vi "AG33XXX.set DC offset.vi"(0 "i ref in":refnum<vi>, 2 "DCOffset [V]":dbl, 3 "ms timeout (10000)":i32=10000, 5 "error in (no error)":errorcluster) -> (14 "i ref out":refnum<vi>, 17 "timed out":bool, 19 "error out":errorcluster)   [LabVIEW 2014, in "AG33XXX.lvlib"]
doc: "Sets the DC offset at my device."
uses:
  AG33XXX.lvlib
  CSCore/CSApplicationBaseClasses/AFGBase/AFGBase.serviceType.ctl
  CSCore/CSApplicationBaseClasses/AFGBase/AFGBase.directionType.ctl
  CSlibraries/UtilityLib/UtilityLib.valueStatus.ctl
  CSCore/CSApplicationBaseClasses/DeviceBase/DeviceBase.lvlib
  CSCore/CSApplicationBaseClasses/AFGBase/AFGBase.lvlib
  CSlibraries/UtilityLib/UtilityLib.lvlib
  CSinstr.lib/Agilent 33xxx Series/Agilent 33XXX Series.lvlib
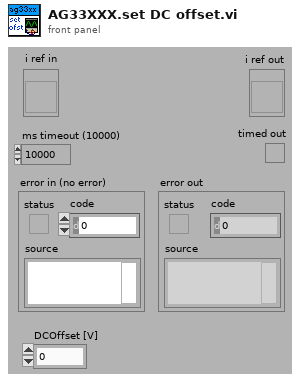
[diagram p1: front panel]
types:
  T1 = typedef "UtilityLib.lvlib/UtilityLib.valueStatus.ctl" = enum16{"no info available", "stand by/off", "on", "warning", "alarm/malfunction", "not implemented", "user action required", "important information", "system default", "control default", "indicator default", "button default"}
  T2 = typedef "AFGBase.lvlib/AFGBase.directionType.ctl" = enum16{"unknown", "update actual value", "update nominal value", "update both"}
  T3 = typedef "AFGBase.lvlib/AFGBase.serviceType.ctl" = enum16{"frequency", "amplitude", "phase", "DCOffset", "enableOutput", "trigger", "waveformType"}
  T4 = typedef "AFGBase.lvlib/AFGBase.i attribute.ctl" = cluster{"actValues":T5, "nomValues":T5}
  T5 = typedef "AFGBase.lvlib/AFGBase.parameters.ctl" = cluster{"frequency":dbl, "amplitude":dbl, "phase":dbl, "DCOffset":dbl, "waveformType":T6, "enableOutput":bool, "trigger":i16[], "serviceIDs":cluster{"frequencyID":i32, "amplitudeID":i32, "phaseID":i32, "DCOffsetID":i32, "waveformTypeID":i32, "enableOutputID":i32, "triggerID":i32}, "waveform":cluster{"data":waveform(dbl), "gain":dbl, "offset":dbl, "repetitionRate":dbl, "sampleRate":dbl}}
  T6 = typedef "AFGBase.lvlib/AFGBase.waveformType.ctl" = enum16{"sine", "square", "ramp", "pulse", "noise", "DC", "arbitrary", "triangle", "ramp_up", "ramp_down", "amplitude modulation"}
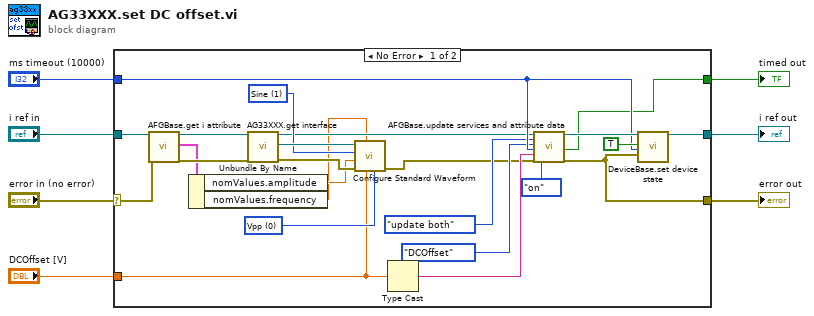
[diagram p0: block diagram]
diagram:
  n1 = case shown="No Error" "error in (no error)" {
    selector: "error in (no error)" -> [w20 w32]
    tunnel: [w31 w33] -> w7
    tunnel: "ms timeout (10000)" -> [w27 _]
    tunnel: "i ref in" -> [w21 w33]
    tunnel: [w28 w32] -> w3
    tunnel: "DCOffset [V]" -> [w10 _]
    tunnel: [w8 _] -> w1
    frame No Error {
      w13 = u16 0 items=["Vpp", "Vrms", "dB"] ("Unit (0: Vpp)")
      w15 = u16 1 items=["DC", "Sine", "Square", "Triangle", "Ramp", "Pulse", "Noise", "Sinc", "Negative Ramp", "Exponential Rise", "Exponential Fall", "Cardiac"] ("Waveform Function (1: Sine)")
      n2 = call "AFGBase.get i attribute.vi"("i ref in"=w21, "error in (no error)"=w20) -> ("i ref out"=w18:refnum<vi>, "i attribute"=w17:T4, "error out"=w19:errorcluster)  [unwired: 15 in]
      n3 = Unbundle By Name(w17) -> ("nomValues.amplitude"=w14:dbl, "nomValues.frequency"=w9:dbl)
      n4 = call "AG33XXX.get interface.vi"("i ref in"=w18, "error in (no error)"=w19) -> ("i ref out"=w11:refnum<vi>, "interface"=w22:refnum<visa-resource-name>, "error out"=w16:errorcluster)  [unwired: 15 in]
      n5 = call "Configure Standard Waveform.vi"("Unit (0: Vpp)"=w13, "DC Offset (0.00 V)"=w10, "Frequency (1000 Hz)"=w9, "error in (no error)"=w16, "Amplitude (1)"=w14, "Waveform Function (1: Sine)"=w15, "VISA resource name"=w22) -> ("error out"=w12:errorcluster)  [unwired: 3 in, 1 out]
      n6 = Type Cast(x=w10) -> (*(type *) &x=w25:string)  [unwired: 1 in]
      n7 = call "AFGBase.update services and attribute data.vi"("i ref in"=w11, "direction"=AFGBase.directionType."update both", "service"=AFGBase.serviceType."DCOffset", "ms timeout (10000)"=w27, "value"=w25, "error in (no error)"=w12, "quality"=UtilityLib.valueStatus."on") -> ("i ref out"=w29:refnum<vi>, "timed out"=w8:bool, "error out"=w28:errorcluster)  [unwired: 10 in]
      n8 = call "DeviceBase.set device state.vi"("i ref in"=w29, "implicit"=TRUE, "ms timeout (10000)"=w27, "device error"=w28) -> ("i ref out"=w31:refnum<vi>)  [unwired: 13 in, 2 out]
    }
    frame Error {
    }
  }
  "error out" <- w3
  "i ref out" <- w7
  "timed out" <- w1
